vi "Get MX Status.vi"(8 "error in (no error)":errorcluster, 11 "VISA resource name":refnum<visa-resource-name>) -> (0 "error out":errorcluster, 1 "Ready?":bool, 2 "Enabled":bool, 3 "VISA resource name out":refnum<visa-resource-name>, 4 "TRG Polarity Positive":bool, 5 "Local?":bool, 6 "TRG External":bool)   [LabVIEW 2020, in "QuPMXdriver.lvlib"]
doc: "Returns status of Remote/Local, Trigger Internal/External, Trigger Polarity Positive/Negative, Enabled/Disabled, Ready yes/no."
uses:
  QuPMXdriver.lvlib
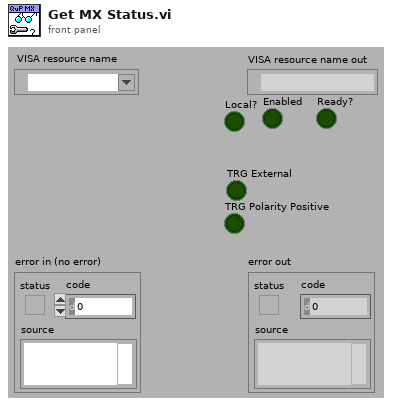
[diagram p1: front panel]
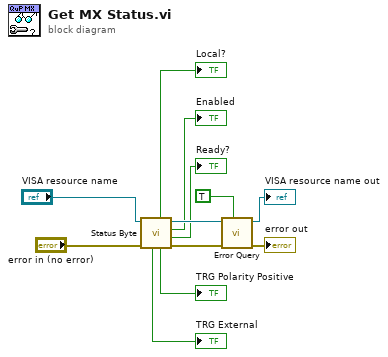
[diagram p0: block diagram]
diagram:
  n1 = call "Status Byte.vi"("error in (no error)"="error in (no error)", "VISA resource name"="VISA resource name") -> ("error out"=w8:errorcluster, "Ready"=→"Ready?":bool, "Enabled"=→"Enabled":bool, "VISA resource name out"=w6:refnum<visa-resource-name>, "TRG Polarity Positive"=→"TRG Polarity Positive":bool, "Local"=→"Local?":bool, "TRG External"=→"TRG External":bool)  [unwired: 2 in, 1 out]
  n2 = call "Error Query.vi"("Ignore empty sequence? (T)"=TRUE, "error in (no error)"=w8, "VISA resource name"=w6) -> ("error out"=→"error out":errorcluster, "VISA resource name out"=→"VISA resource name out":refnum<visa-resource-name>)  [unwired: 7 in]
